vi "Configurate Channel Osciloscope.vi"(8 "error in (no error)":errorcluster, 10 "Configurate Channel--cluster":T1={"Tektronix"={"Enable Channel (True)"=TRUE, "Channel (0: Channel 1)"=0, "Vertical Coupling (1: DC)"=1, "Probe Attenuation (10: 10X)"=10, "Vertical Range (10.0 V/div)"=10.0, "Vertical Offset (0.0 divs)"=0.0, "Bandwidth (0: MAX Bandwidth)"=0}, "EDU-X-1002A"={"Vertical Scale (5.0 V)"=5.0, "Impedance (0: 1 MOhm)"=0, "Channel Name (0: Channel 1)"=0, "Coupling (1: DC)"=1, "Vertical Range (40.0 V)"=40.0, "Vertical Offset (0.0)"=0.0, "Probe Attenuation (1.0)"=1.0, "Vertical Setting (1: Vertical Range)"=1}} {"EDU-X-1002A"."Vertical Setting (1: Vertical Range)" items=["Vertical Scale", "Vertical Range"]; "EDU-X-1002A"."Coupling (1: DC)" items=["AC", "DC"]; "EDU-X-1002A"."Channel Name (0: Channel 1)" items=["Channel 1", "Channel 2", "Channel 3", "Channel 4"]; "EDU-X-1002A"."Impedance (0: 1 MOhm)" items=["1 MOhm", "50 Ohm"]; "Tektronix"."Bandwidth (0: MAX Bandwidth)" items=["MAX Bandwidth", "Unlimited"]; "Tektronix"."Probe Attenuation (10: 10X)" items=["1"=1, "10"=10, "20"=20, "50"=50, "100"=100, "500"=500, "1000"=1000]; "Tektronix"."Vertical Coupling (1: DC)" items=["AC", "DC", "Ground"]; "Tektronix"."Channel (0: Channel 1)" items=["Channel 1", "Channel 2", "Channel 3", "Channel 4", "Math", "Reference A", "Reference B", "Reference C", "Reference D"]}, 11 "Tektronicks in":refnum<class "Tektronicks.lvclass">) -> (0 "error out":errorcluster, 3 "Tektronicks out":refnum<class "Tektronicks.lvclass">)   [LabVIEW 2020, in "Tektronicks.lvclass"]
uses:
  Tektronicks.lvclass
  TypeDefs/ConfigurateCahnnel--cluster.ctl
  Tektronicks.lvclass/Tektronicks.ctl
  <instrlib>/Tektronix TDS 200 1000 2000 Series/Tektronix TDS 200 1000 2000 Series.lvlib
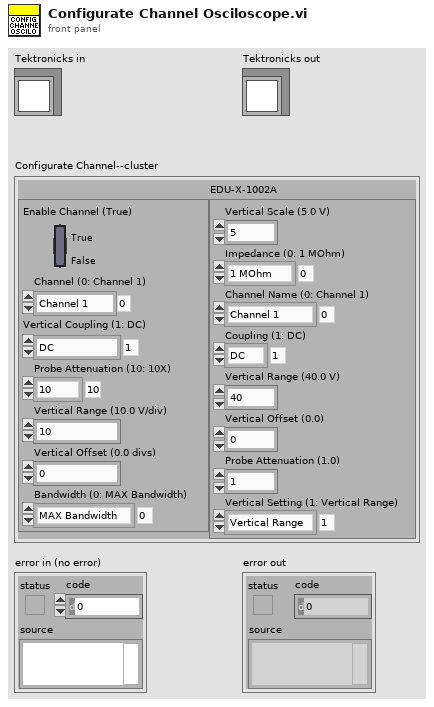
[diagram p1: front panel]
types:
  T1 = typedef "ConfigurateCahnnel--cluster.ctl" = cluster{"Tektronix":cluster{"Enable Channel (True)":bool, "Channel (0: Channel 1)":i32, "Vertical Coupling (1: DC)":i32, "Probe Attenuation (10: 10X)":i32, "Vertical Range (10.0 V/div)":dbl, "Vertical Offset (0.0 divs)":dbl, "Bandwidth (0: MAX Bandwidth)":i32}, "EDU-X-1002A":cluster{"Vertical Scale (5.0 V)":dbl, "Impedance (0: 1 MOhm)":i32, "Channel Name (0: Channel 1)":i32, "Coupling (1: DC)":i32, "Vertical Range (40.0 V)":dbl, "Vertical Offset (0.0)":dbl, "Probe Attenuation (1.0)":dbl, "Vertical Setting (1: Vertical Range)":i32}}
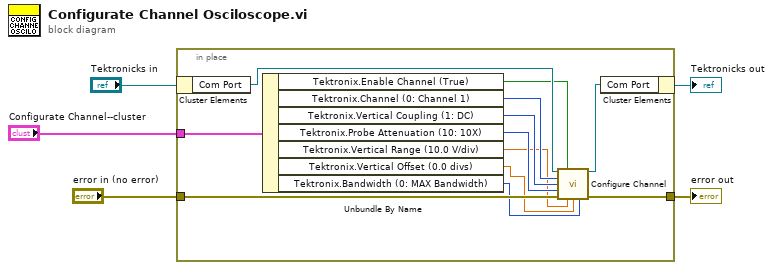
[diagram p0: block diagram]
diagram:
  n1 = in-place {
    in-place-border: [w15] -> w3
    in-place-border: "error in (no error)" -> [w14]
    in-place-border: "Configurate Channel--cluster" -> [w13]
    n2 = in-place-cluster #1("Tektronicks in") -> ("Com Port"=w17:refnum<visa-resource-name>)
    n3 = Unbundle By Name(w13) -> ("Tektronix.Enable Channel (True)"=w12:bool, "Tektronix.Channel (0: Channel 1)"=w11:i32, "Tektronix.Vertical Coupling (1: DC)"=w10:i32, "Tektronix.Probe Attenuation (10: 10X)"=w9:i32, "Tektronix.Vertical Range (10.0 V/div)"=w8:dbl, "Tektronix.Vertical Offset (0.0 divs)"=w7:dbl, "Tektronix.Bandwidth (0: MAX Bandwidth)"=w6:i32)
    n4 = call <instrlib>:"Configure Channel.vi"("VISA resource name"=w17, "Enable Channel (True)"=w12, "Channel (0: Channel 1)"=w11, "Vertical Coupling (1: DC)"=w10, "Probe Attenuation (10: 10X)"=w9, "error in (no error)"=w14, "Vertical Range (10.0 V/div)"=w8, "Vertical Offset (0.0 divs)"=w7, "Bandwidth (0: MAX Bandwidth)"=w6) -> ("VISA resource name out"=w16:refnum<visa-resource-name>, "error out"=w15:errorcluster)  [unwired: 5 in]
    n5 = in-place-cluster #1("Com Port"=w16) -> (→"Tektronicks out":refnum<class "Tektronicks.lvclass">)
  }
  "error out" <- w3
